vi "CANdiSet.vi"   [LabVIEW 2025]
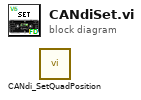
[diagram p0: block diagram]
diagram:
  n1 = call <vilib>:"CANdi_SetQuadPosition.vi"() -> ()  [unwired: 11 in, 1 out]
